vi "Rio_Theta_Position_Sub (DONE).vi"(7 "Desired Position":dbl, 8 "error in (no error)":errorcluster, 11 "Theta Sequence & Position":cluster{i32, dbl}) -> (0 "error out":errorcluster)   [LabVIEW 2017]
doc: "This VI moves the Theta axis from the know position of the limit switch (-120 steps from centre) to a desired input angle. \n\nWritten by Stefan Clarkson, Robin Moore & Thomas Quinn 26/02/18."
uses:
  stepper_half_sequence.ctl
  <vilib>/myRIO/Instrument Drivers/Onboard IO/DIO/typedefs/DIO Reference.ctl
  <vilib>/myRIO/Common/Instrument Driver Framework/Utilities/typedefs/myRIO Generic Hardware Reference.ctl
  <vilib>/myRIO/Common/Instrument Driver Framework/Utilities/typedefs/Hardware Version Enum.ctl
  <vilib>/myRIO/Common/Instrument Driver Framework/Utilities/typedefs/myRIO v1.0 Reference.ctl
  <vilib>/myRIO/Common/Instrument Driver Framework/Utilities/typedefs/Generic FPGA Reference.ctl
  <vilib>/myRIO/Common/Instrument Driver Framework/myRIO v1.0/DIO/typedefs/DIO Channels List.ctl
  <vilib>/myRIO/Common/Instrument Driver Framework/myRIO v1.0/DIO/typedefs/DIO Channels Enum.ctl
  <vilib>/userdefined/High Color/nirio_resource_hc.ctl
  <vilib>/myRIO/Common/Instrument Driver Framework/Utilities/vis/Is FPGA Ref Available.vi
  <vilib>/myRIO/Common/Instrument Driver Framework/myRIO v1.0/DIO/vis/myRIO v1.1 Open DIO.vi
  <vilib>/myRIO/Instrument Drivers/Onboard IO/DIO/vis/Write.vi
  <vilib>/myRIO/Common/Instrument Driver Framework/Utilities/vis/Validate Channels.vi
  <vilib>/myRIO/Common/Instrument Driver Framework/myRIO v1.0/DIO/vis/myRIO v1.0 Reserve DIO.vi
  <vilib>/myRIO/Common/Instrument Driver Framework/myRIO v1.0/Resource Manager/vis/myRIO v1.0 Reserve Channel List.vi
  <vilib>/myRIO/Common/Instrument Driver Framework/myRIO v1.0/DIO/vis/myRIO v1.0 Build MUX Configuration DIO.vi
  <vilib>/myRIO/Common/Instrument Driver Framework/myRIO v1.0/Resource Manager/vis/myRIO v1.0 Reserve Channel.vi
  <vilib>/myRIO/Common/Instrument Driver Framework/myRIO v1.0/Resource Manager/vis/myRIO v1.0 Unreserve Channel.vi
  <vilib>/myRIO/Common/Instrument Driver Framework/myRIO v1.0/Resource Manager/vis/myRIO v1.0 Create Configuration List.vi
  <vilib>/myRIO/Common/Instrument Driver Framework/myRIO v1.0/Resource Manager/vis/myRIO v1.0 Build Mutex Name.vi
  <vilib>/Utility/VariantDataType/GetNumericInfo.vi
  <vilib>/Utility/error.llb/Error Cluster From Error Code.vi
  <vilib>/myRIO/Common/Instrument Driver Framework/myRIO v1.0/myRIO v1.1 Open.vi
  <vilib>/myRIO/Common/Instrument Driver Framework/Utilities/vis/IO Manager.vi
  <vilib>/myRIO/Common/Instrument Driver Framework/Utilities/vis/Configuration Manager.vi
  <vilib>/myRIO/Common/Instrument Driver Framework/myRIO v1.0/Resource Manager/vis/myRIO v1.0 Configure IO.vi
  <vilib>/myRIO/Common/Instrument Driver Framework/myRIO v1.0/myRIO v1.0 Close.vi
  <vilib>/myRIO/Common/Instrument Driver Framework/myRIO v1.0/DIO/vis/myRIO v1.0 Write DIO.vi
  <vilib>/myRIO/Express VI/Onboard IO/DO/DO Express VI.xnode
  <vilib>/myRIO/Instrument Drivers/Onboard IO/DIO/vis/myRIO DIO Open.xnode
  <vilib>/myRIO/Instrument Drivers/Onboard IO/DIO/DIO.lvlib
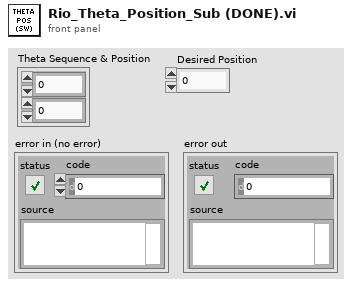
[diagram p1: front panel]
types:
  T1 = typedef "stepper_half_sequence.ctl" = cluster{i32[]}
  T2 = typedef "DIO.lvlib/DIO Reference.ctl" = cluster{"myRIO Reference":T3, "DIO Channels List":T7}
  T3 = typedef "myRIO Generic Hardware Reference.ctl" = cluster{"myRIO Model":T4, "myRIO Hardware Reference":T5}
  T4 = typedef "Hardware Version Enum.ctl" = enum16{"Unknown", "myRIO-1900", "myRIO-1950", "roboRIO", "NI ELVIS RIO CM"}
  T5 = typedef "myRIO v1.0 Reference.ctl" = cluster{"Generic FPGA Reference":T6, "Allow multiple opens":bool}
  T6 = typedef "Generic FPGA Reference.ctl" = refnum<k20>
  T7 = typedef "DIO Channels List.ctl" = T8[]
  T8 = typedef "DIO Channels Enum.ctl" = enum16{"Not Connected", "C/DIO0", "C/DIO1", "C/DIO2", "C/DIO3", "C/DIO4", "C/DIO5", "C/DIO6", "C/DIO7", "A/DIO0", "A/DIO1", "A/DIO2", "A/DIO3", "A/DIO4", "A/DIO5", "A/DIO6", "A/DIO7", "A/DIO8", "A/DIO9", "A/DIO10", "A/DIO11", "A/DIO12", "A/DIO13", "A/DIO14", "A/DIO15", "B/DIO0", "B/DIO1", "B/DIO2", "B/DIO3", "B/DIO4", "B/DIO5", "B/DIO6", "B/DIO7", "B/DIO8", "B/DIO9", "B/DIO10", "B/DIO11", "B/DIO12", "B/DIO13", "B/DIO14", "B/DIO15", "LED0", "LED1", "LED2", "LED3", "Button0", "DIO/DIO0", "DIO/DIO1", "DIO/DIO2", "DIO/DIO3", "DIO/DIO4", "DIO/DIO5", "DIO/DIO6", "DIO/DIO7", "DIO/DIO8", "DIO/DIO9", "SPI/CS0", "SPI/CS1", "SPI/CS2", "SPI/CS3", "LED RADIO (Green)", "LED RADIO (Red)", "LED COMM (Green)", "LED COMM (Red)", "LED MODE (Green)", "LED MODE (Red)"}
  T9 = typedef "nirio_resource_hc.ctl" = tag
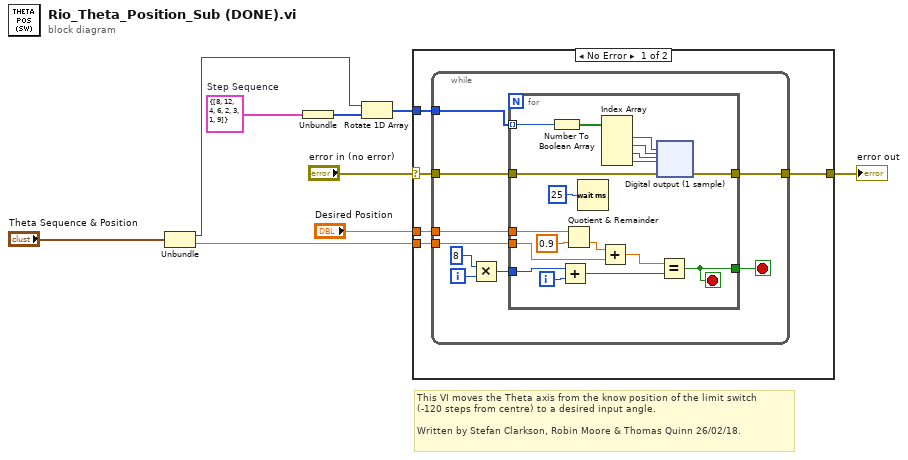
[diagram p0: block diagram]
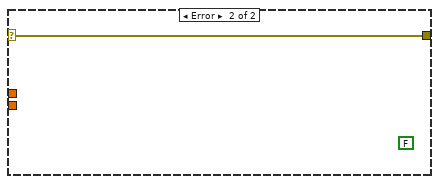
[diagram p2: hidden frame]
diagram:
  w4 = T1 {[8, 12, 4, 6, 2, 3, 1, 9]}  # Step Sequence
  # "This VI moves the Theta axis from the know position of the limit switch \n(-120 steps from centre) to a desired input angle. \n\nWritten by Stefan Clarkson, Robin Moore & Thomas Quinn 26/02/18."
  n1 = Unbundle("Theta Sequence & Position") -> (w8:i32, w9:dbl)
  n2 = Unbundle(w4) -> (w5:i32[])
  n3 = Rotate 1D Array(1:w5, 2:w8) -> (0:w3:i32[])
  n4 = case shown="No Error" "error in (no error)" {
    selector: "error in (no error)" -> [w10 w80]
    tunnel: [w14 w80] -> w2
    tunnel: w3 -> [w13 _]
    tunnel: "Desired Position" -> [w12 _]
    tunnel: w9 -> [w11 _]
    frame No Error {
      n5 = while {
        tunnel: w13 -> [w21]
        tunnel: w10 -> [w22]
        tunnel: [w23] -> w14
        tunnel: w12 -> [w17]
        tunnel: w11 -> [w16]
        i -> [w20]
        stop <- w15 stop-if-true
        n6 = Multiply(x=8, y=w20) -> (x*y=w18:i32)
        n7 = for {
          tunnel: [w35] -> w23
          tunnel: w22 -> [w34]
          tunnel: w21 -> [w33] mode=indexing
          tunnel: w18 -> [w29]
          tunnel: [w26] -> w15
          tunnel: w17 -> [w25]
          tunnel: w16 -> [w24]
          i -> [w28]
          stop <- w26 stop-if-true
          n8 = Number To Boolean Array(number=w33) -> (Boolean array=w41:bool[])
          n9 = Add(x=w29, y=w28) -> (x+y=w27:i32)
          n10 = Quotient & Remainder(x=w25, y=0.9) -> (floor(x/y)=w32:dbl)  [unwired: 1 out]
          n11 = Wait (ms)(milliseconds to wait=u32 25) -> ()  [unwired: 1 out]
          n12 = Add(x=w32, y=w24) -> (x+y=w30:dbl)
          n13 = Index Array(array=w41) -> (element #1=w40:bool, element #2=w39:bool, element #3=w38:bool, element #4=w37:bool)  [unwired: 4 in]
          n14 = xnode ("Digital output (1 sample)")("error in (no error)"=w34, "0 (A/DIO0 (Pin 11))"=w40, "1 (A/DIO1 (Pin 13))"=w39, "2 (A/DIO2 (Pin 15))"=w38, "3 (A/DIO3 (Pin 17))"=w37) -> ("error out"=w35:errorcluster)
          n15 = Equal?(x=w30, y=w27) -> (x = y?=w26:bool)
        }
      }
    }
    frame Error {
      (unwired) FALSE
    }
  }
  "error out" <- w2
